vi "Main.vi"() -> ()   [LabVIEW 2021, in "Application.lvclass"]
uses:
  Application/Application.lvclass
  GameEl_class/private/Enum Direction.ctl
  GameEl_class/GameEl.lvclass
  Snake_class/Snake.lvclass
  Application/Globales Snake.vi
  e26eec9f-965e-4c3b-b51e-9e299e1f8818.vi
  49b93924-5950-4f5a-b15f-497dbc55912f.vi
  Application/Shield.ctl
  Application/Grapes.ctl
  Application/Backgroud_v2.ctl
panel:
  out "Image Ring":u16(ring)
  out "Star":bool
  in  "Grapes":T1
  in  "Shield":T2
  in  "Studios":bool caption="Creator 2"
  in  "Creator":bool
  out "TIME":string
  out "SCORE":string
  out "Board Game":u32[][](array[colorbox])
  out "Background":T3=1
  in  "Usert Stop Game":bool
  in  "Pause/Resume":bool
  out "Direction":T4
  out "Current Score":u16
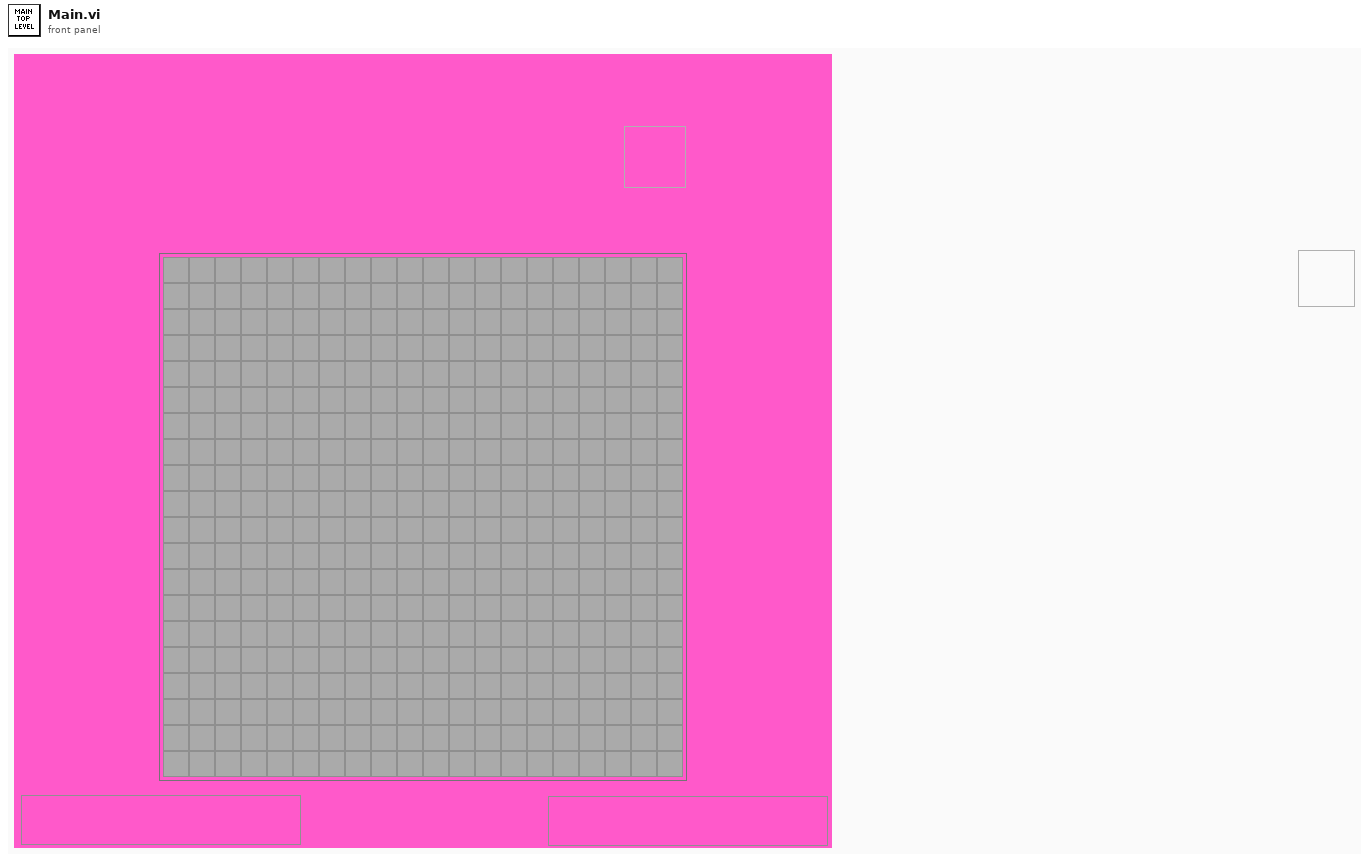
[diagram p1: front panel]
types:
  T1 = typedef "Application.lvclass/Grapes.ctl" = u16
  T2 = typedef "Application.lvclass/Shield.ctl" = u16
  T3 = typedef "Application.lvclass/Backgroud_v2.ctl" = u16
  T4 = typedef "GameEl.lvclass/Enum Direction.ctl" = enum16{"Up", "Down", "Forward", "Backward"}
  T5 = enum8{"Enabled", "Disabled", "Disabled and Grayed Out"}
  T6 = cluster{"Event Registration Refnum":refnum<event-registration>}
  T7 = enum32{"invalid app kind", "Development System", "Run Time System", "Student Edition", "Embedded LabVIEW", "Evaluation", "Custom"}
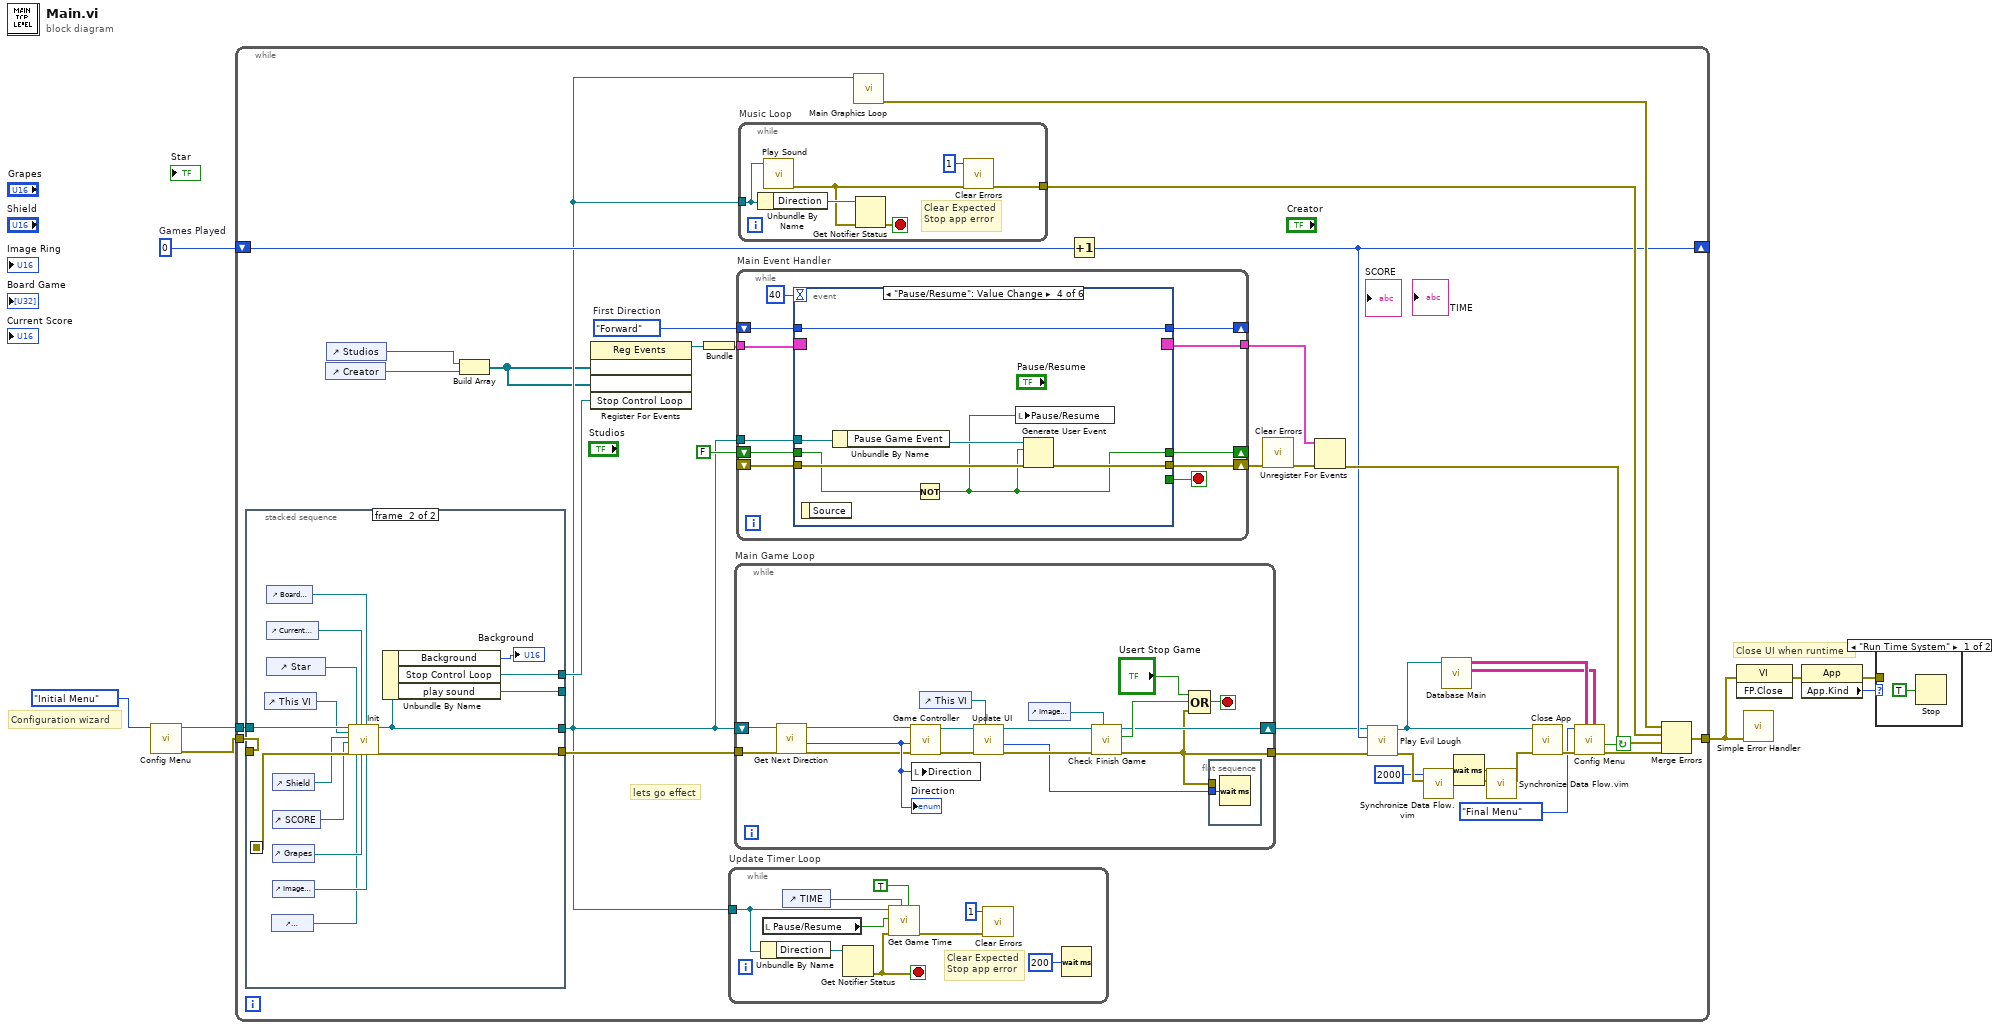
[diagram p0: block diagram]
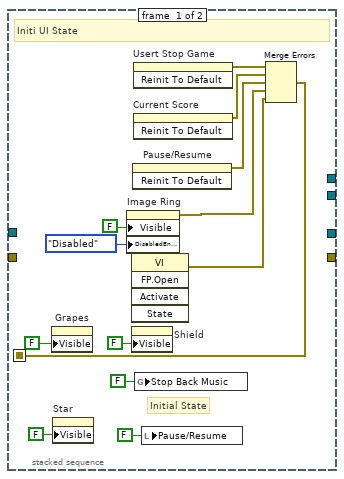
[diagram p2: hidden frame]
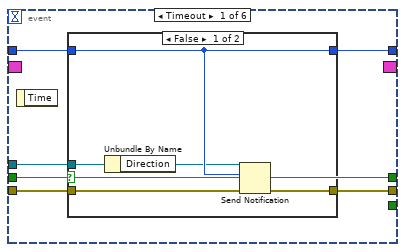
[diagram p3: hidden frame]
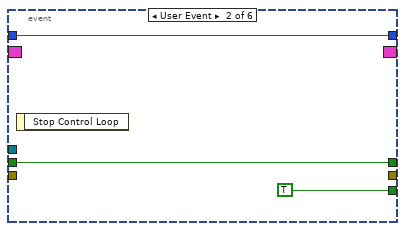
[diagram p5: hidden frame]
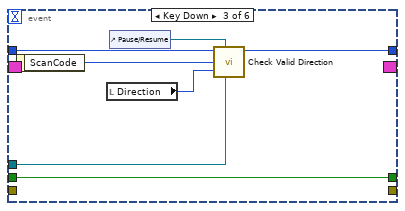
[diagram p6: hidden frame]
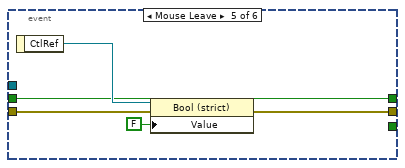
[diagram p7: hidden frame]
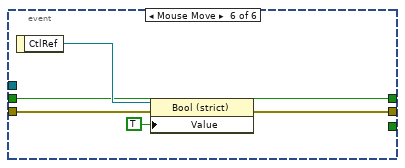
[diagram p8: hidden frame]
diagram:
  w6 = 0  # Games Played
  # "Close UI when runtime"
  # "Configuration wizard"
  n1 = call "Config Menu.vi"("Enum"=enum16{"Initial Menu", "Final Menu"}."Initial Menu") -> ("error out"=w8:errorcluster, "output cluster"=w7:refnum<class "Application.lvclass">)  [unwired: 8 in, 1 out]
  n2 = while {
    tunnel: w8 -> [w34]
    tunnel: [w35] -> w2
    tunnel: w7 -> [w32]
    shift-right: [w30] -> _
    shift-left: w6 -> [w31]
    stop <- w25 continue-if-true
    w43 = Enum_Direction."Forward"  # First Direction
    # "lets go effect"
    n3 = stacked-sequence {
      seq-local: [w80 _] -> [_ w100]
      tunnel: [_ w99] -> w20
      tunnel: [_ w98] -> w17
      tunnel: [_ w95] -> w36
      tunnel: w34 -> [_ _]
      tunnel: w32 -> [_ w90]
      tunnel: [_ w87] -> _
      frame #0 {
        # "Initial State"
        # "Initi UI State"
        n4 = property on="Grapes" class="Ring (strict)"("Visible"=FALSE) -> ()  [unwired: 2 in, 2 out]
        n5 = property on="Star" class="Bool (strict)"("Visible"=FALSE) -> ()  [unwired: 2 in, 2 out]
        n6 = property on="Image Ring" class="Ring (strict)"("Visible"=FALSE, "DisabledEnum"=T5."Disabled" ("Disabled")) -> (error out=w76:errorcluster)  [unwired: 2 in, 1 out]
        n7 = invoke class="VI" method="FP.Open"() -> (error out=w81:errorcluster)  [unwired: 5 in, 4 out]
        n8 = property on="Shield" class="Ring (strict)"("Visible"=FALSE) -> ()  [unwired: 2 in, 2 out]
        n9 = invoke on="Pause/Resume" class="Bool (strict)" method="Reinit To Default"() -> (error out=w82:errorcluster)  [unwired: 3 in, 2 out]
        n10 = invoke on="Usert Stop Game" class="Bool (strict)" method="Reinit To Default"() -> (error out=w84:errorcluster)  [unwired: 3 in, 2 out]
        n11 = invoke on="Current Score" class="DigNum (strict)" method="Reinit To Default"() -> (error out=w83:errorcluster)  [unwired: 3 in, 2 out]
        n12 = global write "Globales Snake.vi" "Stop Back Music"(FALSE ("Stop Back Music")) -> ()
        n13 = local write "Pause/Resume"(FALSE ("Pause/Resume")) -> ()
        n14 = Merge Errors(w84, w83, w82, w76, w81) -> (w80:errorcluster)
      }
      frame #1 {
        n15 = control-ref of="This VI"() -> (w85:refnum<vi>)
        n16 = control-ref of="Board Game"() -> (w97:refnum<vi>)
        n17 = control-ref of="Current Score"() -> (w96:refnum<vi>)
        n18 = control-ref of="Star"() -> (w86:refnum<vi>)
        n19 = control-ref of="Background"() -> (w89:refnum<vi>)
        n20 = control-ref of="Shield"() -> (w94:refnum<vi>)
        n21 = control-ref of="SCORE"() -> (w93:refnum<vi>)
        n22 = control-ref of="Grapes"() -> (w92:refnum<vi>)
        n23 = control-ref of="Image Ring"() -> (w91:refnum<vi>)
        n24 = call "Init.vi"("input cluster"=w90, "This VI"=w85, "Shield"=w94, "SCORE"=w93, "error in (no error)"=w100, "STAR"=w86, "Background"=w89, "Score"=w96, "Grapes"=w92, "Board Game"=w97, "Image Ring"=w91) -> ("Application out"=w98:refnum<class "Application.lvclass">, "error out"=w99:errorcluster)  [unwired: 7 in]
        n25 = Unbundle By Name(w98) -> ("Background"=→"Background":u16, "Stop Control Loop"=w95:refnum<user-event>, "play sound"=w87:refnum<user-event>)
      }
    }
    n26 = control-ref of="Creator"() -> (w19:refnum<vi>)
    n27 = control-ref of="Studios"() -> (w18:refnum<vi>)
    n28 = Build Array(w18, w19) -> (w16:refnum<vi>[])
    n29 = register-events(w16, w16, w36) -> (reference out=w44:refnum<event-registration>)  [unwired: 2 in, 1 out]
    n30 = Bundle("Event Registration Refnum"=w44) -> (w21:T6)  [unwired: 1 in]
    n31 = while "Update Timer Loop" {
      tunnel: w17 -> [w70]
      stop <- w68 stop-if-true
      # "Clear Expected\nStop app error"
      n32 = Unbundle By Name(w70) -> ("Direction"=w69:refnum<notifier>)
      n33 = local read "Pause/Resume"() -> (w65:bool)
      n34 = control-ref of="TIME"() -> (w64:refnum<vi>)
      n35 = Get Notifier Status(notifier=w69) -> (error out=w68:errorcluster)  [unwired: 1 in, 4 out]
      n36 = call "Get Game Time.vi"("update ui"=TRUE, "Time"=w64, "error in (no error)"=w68, "Pause/Resume"=w65, "Application in"=w70) -> ("error out"=w66:errorcluster)  [unwired: 4 in, 2 out]
      n37 = call <vilib>:"Clear Errors.vi"("error in (no error)"=w66, "specific error code to clear (0: all)"=1) -> ()  [unwired: 4 in, 2 out]
      n38 = Wait (ms)(milliseconds to wait=u32 200) -> ()  [unwired: 1 out]
    }
    n39 = while "Main Game Loop" {
      tunnel: w20 -> [w54]
      tunnel: [w46] -> w28
      shift-right: [w50] -> w29
      shift-left: w17 -> [w59]
      stop <- w61 stop-if-true
      n40 = call "Get Next Direction.vi"("error in (no error)"=w54, "Application in"=w59) -> ("error out"=w49:errorcluster, "Direction"=w56:T4, "Application out"=w58:refnum<class "Application.lvclass">)  [unwired: 7 in]
      "Direction" <- w56
      n41 = call "Game Controller.vi"("error in (no error)"=w49, "Direction"=w56, "Application in"=w58) -> ("error out"=w52:errorcluster, "Application out"=w53:refnum<class "Application.lvclass">)  [unwired: 7 in]
      n42 = local write "Direction"(w56) -> ()
      n43 = control-ref of="This VI"() -> (w47:refnum<vi>)
      n44 = call "Update UI.vi"("This VI"=w47, "error in (no error)"=w52, "Application in"=w53) -> ("error out"=w48:errorcluster, "Time"=w45:u32, "Application out"=w51:refnum<class "Application.lvclass">)  [unwired: 6 in]
      n45 = control-ref of="Image Ring"() -> (w57:refnum<vi>)
      n46 = call "Check Finish Game.vi"("Game Result"=w57, "error in (no error)"=w48, "Application in"=w51) -> ("error out"=w46:errorcluster, "Finish Game?"=w55:bool, "Application out"=w50:refnum<class "Application.lvclass">)  [unwired: 6 in]
      n47 = Compound Arithmetic op=OR("Usert Stop Game", w55, w46) -> (w61:bool)
      n48 = flat-sequence {
        tunnel: w46 -> [_]
        tunnel: w45 -> [w62]
        frame #0 {
          n49 = Wait (ms)(milliseconds to wait=w62) -> ()  [unwired: 1 out]
        }
      }
    }
    n50 = while "Main Event Handler" {
      tunnel: w21 -> [w117]
      tunnel: [w115] -> w39
      shift-right: [w113] -> _
      shift-left: w43 -> [w111]
      tunnel: w17 -> [w112]
      shift-right: [w109] -> w41
      shift-left: _ -> [w110]
      shift-right: [w107] -> _
      shift-left: FALSE -> [w108]
      stop <- w116 stop-if-true
      n51 = event shown="[3] \"Pause/Resume\": Value Change" {
        selector: w117 -> [_ _ _ _ _ _]
        dyn-events: [_ _ _ _ _ _] -> w115
        timeout: 40 -> [_ _ _ _ _ _]
        tunnel: [_ TRUE _ _ _ _] -> w116
        tunnel: [w119 w132 w138 w147 _ _] -> w113
        tunnel: w112 -> [w123 _ w134 w144 _ _]
        tunnel: w111 -> [w120 w132 w139 w147 _ _]
        tunnel: w110 -> [w121 _ _ w146 w152 w157]
        tunnel: [w122 _ _ w145 w151 w156] -> w109
        tunnel: w108 -> [w118 w131 w140 w142 w148 w153]
        tunnel: [w118 w131 w140 w141 w148 w153] -> w107
        event Timeout {
          n52 = event-data() -> ()  [unwired: 1 in, 1 out]
          n53 = case shown="False" w118 {
            tunnel: w123 -> [w128 _]
            tunnel: [w127 w129] -> w122
            tunnel: w121 -> [w126 w129]
            tunnel: w120 -> [w125 w130]
            tunnel: [w125 w130] -> w119
            frame False {
              n54 = Unbundle By Name(w128) -> ("Direction"=w124:refnum<notifier>)
              n55 = Send Notification(notification=w125, notifier=w124, error in (no error)=w126) -> (error out=w127:errorcluster)  [unwired: 1 out]
            }
            frame True {
            }
          }
        }
        event User Event {
          n56 = event-data() -> ()  [unwired: 1 in, 1 out]
        }
        event Key Down {
          n57 = event-data() -> ("ScanCode"=w136:i16)  [unwired: 1 in]
          n58 = local read "Direction"() -> (w137:T4)
          n59 = control-ref of="Pause/Resume"() -> (w135:refnum<vi>)
          n60 = call "Check Valid Direction.vi"("Application out"=w134, "Pause/Resume Ref"=w135, "Last Movement"=w137, "ScanCode"=w136, "Current Direction"=w139) -> ("New Direction"=w138:T4)  [unwired: 6 in]
        }
        event "Pause/Resume": Value Change {
          n61 = event-data() -> ()  [unwired: 1 in, 1 out]
          n62 = Unbundle By Name(w144) -> ("Pause Game Event"=w143:refnum<user-event>)
          n63 = Not(x=w142) -> (.not. x?=w141:bool)
          n64 = local write "Pause/Resume"(w141) -> ()
          n65 = Generate User Event(user event=w143, event data cluster=w141, error in=w146) -> (error out=w145:errorcluster)  [unwired: 1 in, 1 out]
        }
        event Mouse Leave {
          n66 = event-data() -> ("CtlRef"=w150:refnum<vi>)  [unwired: 1 in]
          n67 = property class="Bool (strict)"(reference=w150, error in=w152, "Value"=FALSE) -> (error out=w151:errorcluster)  [unwired: 1 out]
        }
        event Mouse Move {
          n68 = event-data() -> ("CtlRef"=w155:refnum<vi>)  [unwired: 1 in]
          n69 = property class="Bool (strict)"(reference=w155, error in=w157, "Value"=TRUE) -> (error out=w156:errorcluster)  [unwired: 1 out]
        }
      }
    }
    n70 = while "Music Loop" {
      tunnel: [w104] -> w37
      tunnel: w17 -> [w102]
      stop <- w105 stop-if-true
      # "Clear Expected\nStop app error"
      n71 = Unbundle By Name(w102) -> ("Direction"=w106:refnum<notifier>)
      n72 = call "Play Sound.vi"("Application In"=w102) -> ("error out"=w101:errorcluster)  [unwired: 10 in]
      n73 = Get Notifier Status(notifier=w106, error in (no error)=w101) -> (error out=w105:errorcluster)  [unwired: 4 out]
      n74 = call <vilib>:"Clear Errors.vi"("error in (no error)"=w101, "specific error code to clear (0: all)"=1) -> ("error out"=w104:errorcluster)  [unwired: 4 in, 1 out]
    }
    n75 = call "Main Graphics Loop.vi"("Application in"=w17) -> ("error out"=w33:errorcluster)  [unwired: 10 in]
    n76 = Increment(x=w31) -> (x+1=w30:i32)
    n77 = call <vilib>:"Clear Errors.vi"("error in (no error)"=w41) -> ("error out"=w40:errorcluster)  [unwired: 5 in, 1 out]
    n78 = Unregister For Events(event registration refnum=w39, error in=w40) -> (error out=w38:errorcluster)
    n79 = call "Play Evil Lough.vi"("error in (no error)"=w28, "Number of games"=w30, "Application in"=w29) -> ("error out"=w14:errorcluster, "Application out"=w23:refnum<class "Application.lvclass">)  [unwired: 7 in]
    n80 = call "Synchronize Data Flow.vim"("input 2"=w14, "input 1"=u32 2000 ("milliseconds to wait")) -> ("output 2"=w11:errorcluster, "output 1"=w12:u32)  [unwired: 2 in, 2 out]
    n81 = call "Database Main.vi"("Application.lvclass"=w23) -> ("Stats"=w15:string[][], "Games"=w22:string[][])  [unwired: 9 in]
    n82 = Wait (ms)(milliseconds to wait=w12) -> (millisecond timer value=w10:u32)
    n83 = call "Synchronize Data Flow.vim"("input 2"=w11, "input 1"=w10) -> ("output 2"=w9:errorcluster)  [unwired: 2 in, 3 out]
    n84 = call "Close App.vi"("error in (no error)"=w9, "Application in"=w23) -> ("error out"=w27:errorcluster)  [unwired: 9 in]
    n85 = call "Config Menu.vi"("Stats"=w15, "Data Out"=w22, "error in (no error)"=w27, "Enum"=enum16{"Initial Menu", "Final Menu"}."Final Menu") -> ("error out"=w24:errorcluster, "Play/stop"=w25:bool)  [unwired: 5 in, 1 out]
    n86 = Merge Errors(w33, w37, w38, w24) -> (w35:errorcluster)
  }
  n87 = invoke class="VI" method="FP.Close"(error in=w2) -> (error out=w1:errorcluster)  [unwired: 2 in, 2 out]
  n88 = call <vilib>:"Simple Error Handler.vi"("error in (no error)"=w2) -> ()  [unwired: 4 in, 5 out]
  n89 = property class="App"(error in=w1) -> (error out=w3:errorcluster, "App.Kind"=w4:T7)  [unwired: 1 in, 1 out]
  n90 = case shown="\"Run Time System\"" w4 {
    tunnel: w3 -> [_ _]
    frame "Run Time System" {
      n91 = Stop(stop? (T)=TRUE) -> ()
    }
    frame Default {
    }
  }
